vi "PH_ImageOperator.write PSDB Cam Settings data.vi"(0 "i ref in":refnum<vi>, 5 "error in":errorcluster) -> (14 "i ref out":refnum<vi>, 16 "Cam Settings Boolean data":T3[](array[typedef]), 17 "Cam Settings Numeric data":T2[](array[typedef]), 18 "Cam Settings String data":T1[](array[typedef]), 19 "error out":errorcluster)   [LabVIEW 2014, in "PH_ImageOperator.lvlib"]
uses:
  PH_ImageOperator.lvlib
  PH_PSDBWriter/PH_PSDBWriter.Boolean dataset.ctl
  PH_PSDBWriter/PH_PSDBWriter.Numeric dataset.ctl
  PH_PSDBWriter/PH_PSDBWriter.String dataset.ctl
  PH_Img_BaseClass/PH_Img_BaseClass.lvlib
  PH_PSDBWriter/PH_PSDBWriter.lvlib
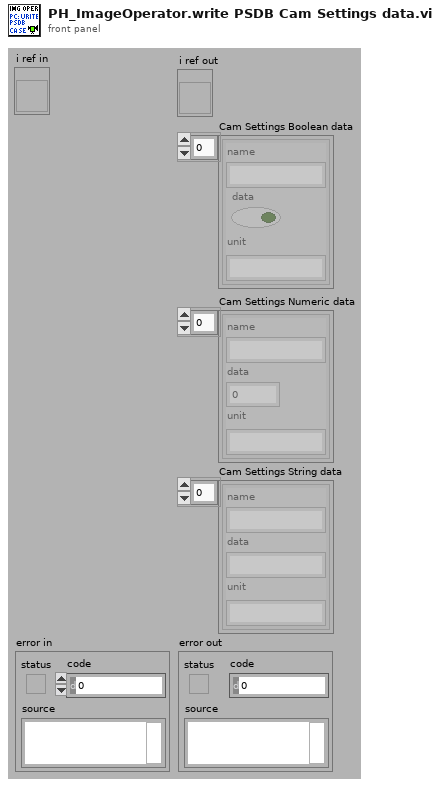
[diagram p1: front panel]
types:
  T1 = typedef "PH_PSDBWriter.lvlib/PH_PSDBWriter.String dataset.ctl" = cluster{"name":string, "data":string, "unit":string}
  T2 = typedef "PH_PSDBWriter.lvlib/PH_PSDBWriter.Numeric dataset.ctl" = cluster{"name":string, "data":dbl, "unit":string}
  T3 = typedef "PH_PSDBWriter.lvlib/PH_PSDBWriter.Boolean dataset.ctl" = cluster{"name":string, "data":bool, "unit":string}
  T4 = typedef "PH_Img_BaseClass.lvlib/PH_Img_BaseClass.i attribute.ctl" = cluster{"GUI Refs":T5, "Timeout Image [ms]":i32, "Default Periodic Period [ms]":i32, "Camera":cluster{"Instancename":string, "Notifier":refnum<notifier>}, "Palette":T6, "Cam Settings":cluster{"Cam ID":string, "Gain":dbl, "Brightness":dbl, "Shutter":dbl, "Cam Info Failure":bool, "Mode":i32}}
  T5 = typedef "PH_Img_BaseClass.lvlib/PH_Img_BaseClass.GUI Refs.ctl" = cluster{"Timeout":refnum<vi>, "Image":refnum<vi>, "Palette":refnum<vi>, "Timeout Set":refnum<vi>}
  T6 = typedef "PH_Img_BaseClass.lvlib/PH_Img_BaseClass.Palette.ctl" = i32
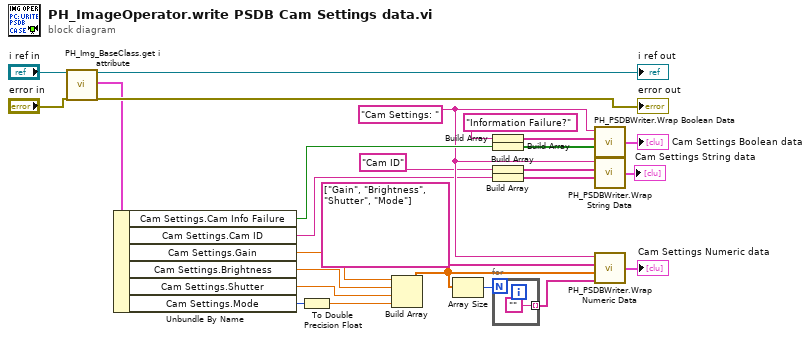
[diagram p0: block diagram]
diagram:
  w4 = "Cam Settings: " ("string")
  n1 = call "PH_Img_BaseClass.get i attribute.vi"("i ref in"="i ref in", "error in (no error)"="error in") -> ("i ref out"=→"i ref out":refnum<vi>, "i attribute"=w20:T4, "error out"=→"error out":errorcluster)  [unwired: 15 in]
  n2 = Unbundle By Name(w20) -> ("Cam Settings.Cam Info Failure"=w14:bool, "Cam Settings.Cam ID"=w3:string, "Cam Settings.Gain"=w9:dbl, "Cam Settings.Brightness"=w8:dbl, "Cam Settings.Shutter"=w7:dbl, "Cam Settings.Mode"=w22:i32)
  n3 = To Double Precision Float(number=w22) -> (double precision float=w21:dbl)
  n4 = Build Array(w9, w8, w7, w21) -> (w17:dbl[])
  n5 = Array Size(array=w17) -> (size(s)=w18:i32)
  n6 = Build Array("Information Failure?" ("string")) -> (w11:string[])
  n7 = Build Array(w14) -> (w10:bool[])
  n8 = Build Array("Cam ID") -> (w6:string[])
  n9 = Build Array(w3) -> (w5:string[])
  n10 = for {
    N: w18 -> [_]
    tunnel: [""] -> w16 mode=indexing
  }
  n11 = call "PH_PSDBWriter.Wrap Boolean Data.vi"("Data Array"=w10, "Name Array"=w11, "Name Prefix"=w4) -> ("PSDB Boolean Data Array"=→"Cam Settings Boolean data":T3[])  [unwired: 1 in]
  n12 = call "PH_PSDBWriter.Wrap String Data.vi"("Data Array"=w5, "Name Array"=w6, "Name Prefix"=w4) -> ("PSDB String Data Array"=→"Cam Settings String data":T1[])  [unwired: 1 in]
  n13 = call "PH_PSDBWriter.Wrap Numeric Data.vi"("Unit Array"=w16, "Data Array"=w17, "Name Array"=string[] ["Gain", "Brightness", "Shutter", "Mode"], "Name Prefix"=w4) -> ("PSDB Numeric Data Array"=→"Cam Settings Numeric data":T2[])
